vi "Teleop.vi"(10 "Match Info":T1={"Autonomous Elapsed Seconds"=0.0, "TeleOp Elapsed Seconds"=0.0, "Disabled Elapsed Seconds"=0.0, "Visited Autonomous"=FALSE, "Visited TeleOp"=FALSE, "Visited Disabled"=FALSE, "Autonomous Settings"={"Autonomous Style"=enum."Independent", "VI Refnum"=refnum}}, 11 "Call Context":T2) -> ()   [LabVIEW 2018]
doc: "This VI is called for each TeleOp packet received from the DS where the robot is not disabled. It is often used to read from the joysticks and update I/O or to update setpoints for timed control loops. It should complete and return within 20 milliseconds or it may miss DS packets."
uses:
  <vilib>/Rock Robotics/WPI/DriverStation/WPI_DriverStationDerivedRobotMode.ctl
  <vilib>/Rock Robotics/WPI/DriverStation/WPI_DriverStationMatch Info.ctl
  <vilib>/Rock Robotics/WPI/Solenoid/WPI_SolenoidValue.ctl
  <vilib>/Rock Robotics/WPI/ThirdParty/Phoenix-LabVIEW/Motor Controller/Controls/CTRE_Phoenix_MotorControl_ControlMode.ctl
  069bde93-6a50-4702-a448-63a100da85ba.vi
  93fe4f39-d887-44e8-b42b-40b0db67de57.vi
  <vilib>/Rock Robotics/WPI/Utilities/WPI_GetSetVariantRefNum.vi
  <vilib>/Rock Robotics/Network Tables/NT Write Boolean Array.vi
  <vilib>/Rock Robotics/Network Tables/NT Write Numeric Array.vi
  <vilib>/Rock Robotics/Network Tables/NT Read Boolean.vi
  <vilib>/Rock Robotics/Network Tables/NT Read Number.vi
  Robot Global Data.vi
  <vilib>/Rock Robotics/WPI/Solenoid/WPI_SolenoidSetEnum.vi
  <vilib>/Rock Robotics/WPI/ThirdParty/Phoenix-LabVIEW/Motor Controller/Get/CTRE_Phoenix_MotorController_GetSelectedSensorData.vi
  <vilib>/Rock Robotics/WPI/ThirdParty/Phoenix-LabVIEW/Motor Controller/Get/CTRE_Phoenix_MotorController_GetOutputCurrent_Enhanced.vi
panel:
  out "Level":string="Low"
  out "GamePiece":string="Hatch"
  out "Output Voltage 4":dbl
  out "Output Voltage 3":dbl
  out "Output Voltage 2":dbl
  out "Output Voltage":dbl
  out "wrist sensor":i32
  out "Arm sensor":i32
  out "x output 2":dbl
  out "y output 2":dbl
  out "Sample Slider 0":dbl(slide) scale=0.0..5.0
  out "Sample Boolean 1":bool
  out "Sample Boolean 0":bool
  # "left"
  # "RIGHT"
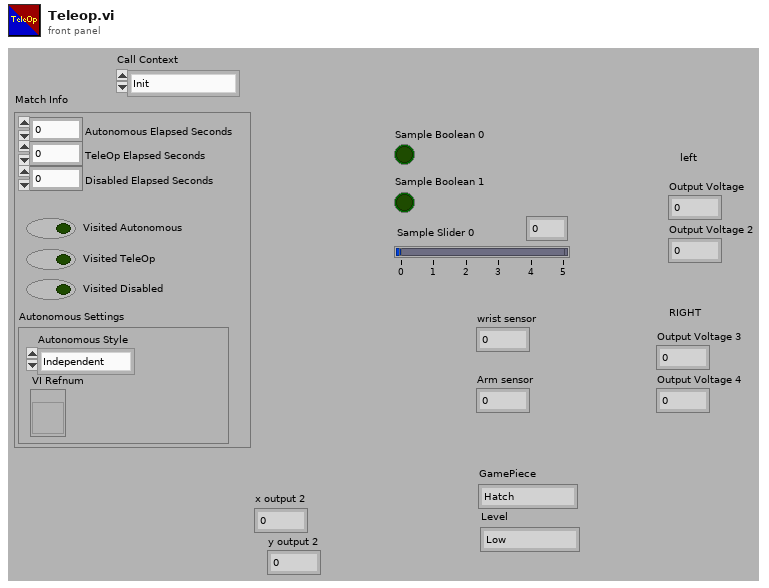
[diagram p1: front panel]
types:
  T1 = typedef "WPI_DriverStationMatch Info.ctl" = cluster{"Autonomous Elapsed Seconds":dbl, "TeleOp Elapsed Seconds":dbl, "Disabled Elapsed Seconds":dbl, "Visited Autonomous":bool, "Visited TeleOp":bool, "Visited Disabled":bool, "Autonomous Settings":cluster{"Autonomous Style":enum16{"Iterative", "Independent"}, "VI Refnum":refnum<vi>}}
  T2 = typedef "WPI_DriverStationDerivedRobotMode.ctl" = enum16{"Init", "Execute", "Stop"}
  T3 = typedef "WPI_SolenoidValue.ctl" = enum16{"Off", "On", "Forward", "Reverse"}
  T4 = typedef "WPI_JoystickDevRef.ctl" = cluster{"Device":T5}
  T5 = typedef "WPI_JoystickDeviceEnum.ctl" = enum16{"USB 0", "USB 1", "USB 2", "USB 3", "USB 4", "USB 5"}
  T6 = typedef "WPI_RobotDriveDevRef.ctl" = cluster{"DevStatus":errorcluster, "Motors[]":T7[], "Square Inputs":bool, "Max Output":dbl}
  T7 = typedef "WPI_MotorControlDeviceRef.ctl" = cluster{"DeviceStatus":errorcluster, "Type":T8, "PWM":cluster{"PWM Channel":T9, "DeadBand":T10}, "CAN":cluster{"Device Number":u8, "SetOutput VI Ref":variant, "GetOutput VI Ref":variant, "Enable VI Ref":variant, "Disable VI Ref":variant, "Data":variant}, "Invert":bool, "DIO PWM":cluster{"PWM \"Enable\" Channel":T9, "DIOChannel":T11, "PWM Rate":dbl}}
  T8 = typedef "WPI_MotorControlType.ctl" = enum16{"PWM", "CAN", "DIO PWM"}
  T9 = typedef "FPGA_DIOPWMChannel.ctl" = enum8{"PWM 0", "PWM 1", "PWM 2", "PWM 3", "PWM 4", "PWM 5", "PWM 6", "PWM 7", "PWM 8", "PWM 9", "PWM MXP 0", "PWM MXP 1", "PWM MXP 2", "PWM MXP 3", "PWM MXP 4", "PWM MXP 5", "PWM MXP 6", "PWM MXP 7", "PWM MXP 8", "PWM MXP 9", "Invalid"}
  T10 = typedef "WPI_PWMDeadband.ctl" = cluster{"Name":string, "maxPositivePwm":i32, "minPositivePwm":i32, "centerPwm":i32, "maxNegativePwm":i32, "minNegativePwm":i32, "angularRange":u16}
  T11 = typedef "FPGA_DIOChannel.ctl" = enum8{"DIO 0", "DIO 1", "DIO 2", "DIO 3", "DIO 4", "DIO 5", "DIO 6", "DIO 7", "DIO 8", "DIO 9", "DIO MXP 0", "DIO MXP 1", "DIO MXP 2", "DIO MXP 3", "DIO MXP 4", "DIO MXP 5", "DIO MXP 6", "DIO MXP 7", "DIO MXP 8", "DIO MXP 9", "DIO MXP 10", "DIO MXP 11", "DIO MXP 12", "DIO MXP 13", "DIO MXP 14", "DIO MXP 15", "SPI Port CS1", "SPI Port CS2", "SPI Port CS3", "SPI Port MISO", "SPI Port MOSI", "Invalid"}
  T12 = typedef "WPI_SolenoidDevRef.ctl" = cluster{"DevStatus":errorcluster, "Pneumatics Control Module":u8, "Forward Solenoid Channel":T13, "Reverse Solenoid Channel":T13}
  T13 = typedef "WPI_SolenoidChannel.ctl" = enum8{"Solenoid 0", "Solenoid 1", "Solenoid 2", "Solenoid 3", "Solenoid 4", "Solenoid 5", "Solenoid 6", "Solenoid 7", "Invalid"}
  T14 = typedef "CTRE_Phoenix_MotorControl_ControlMode.ctl" = u16
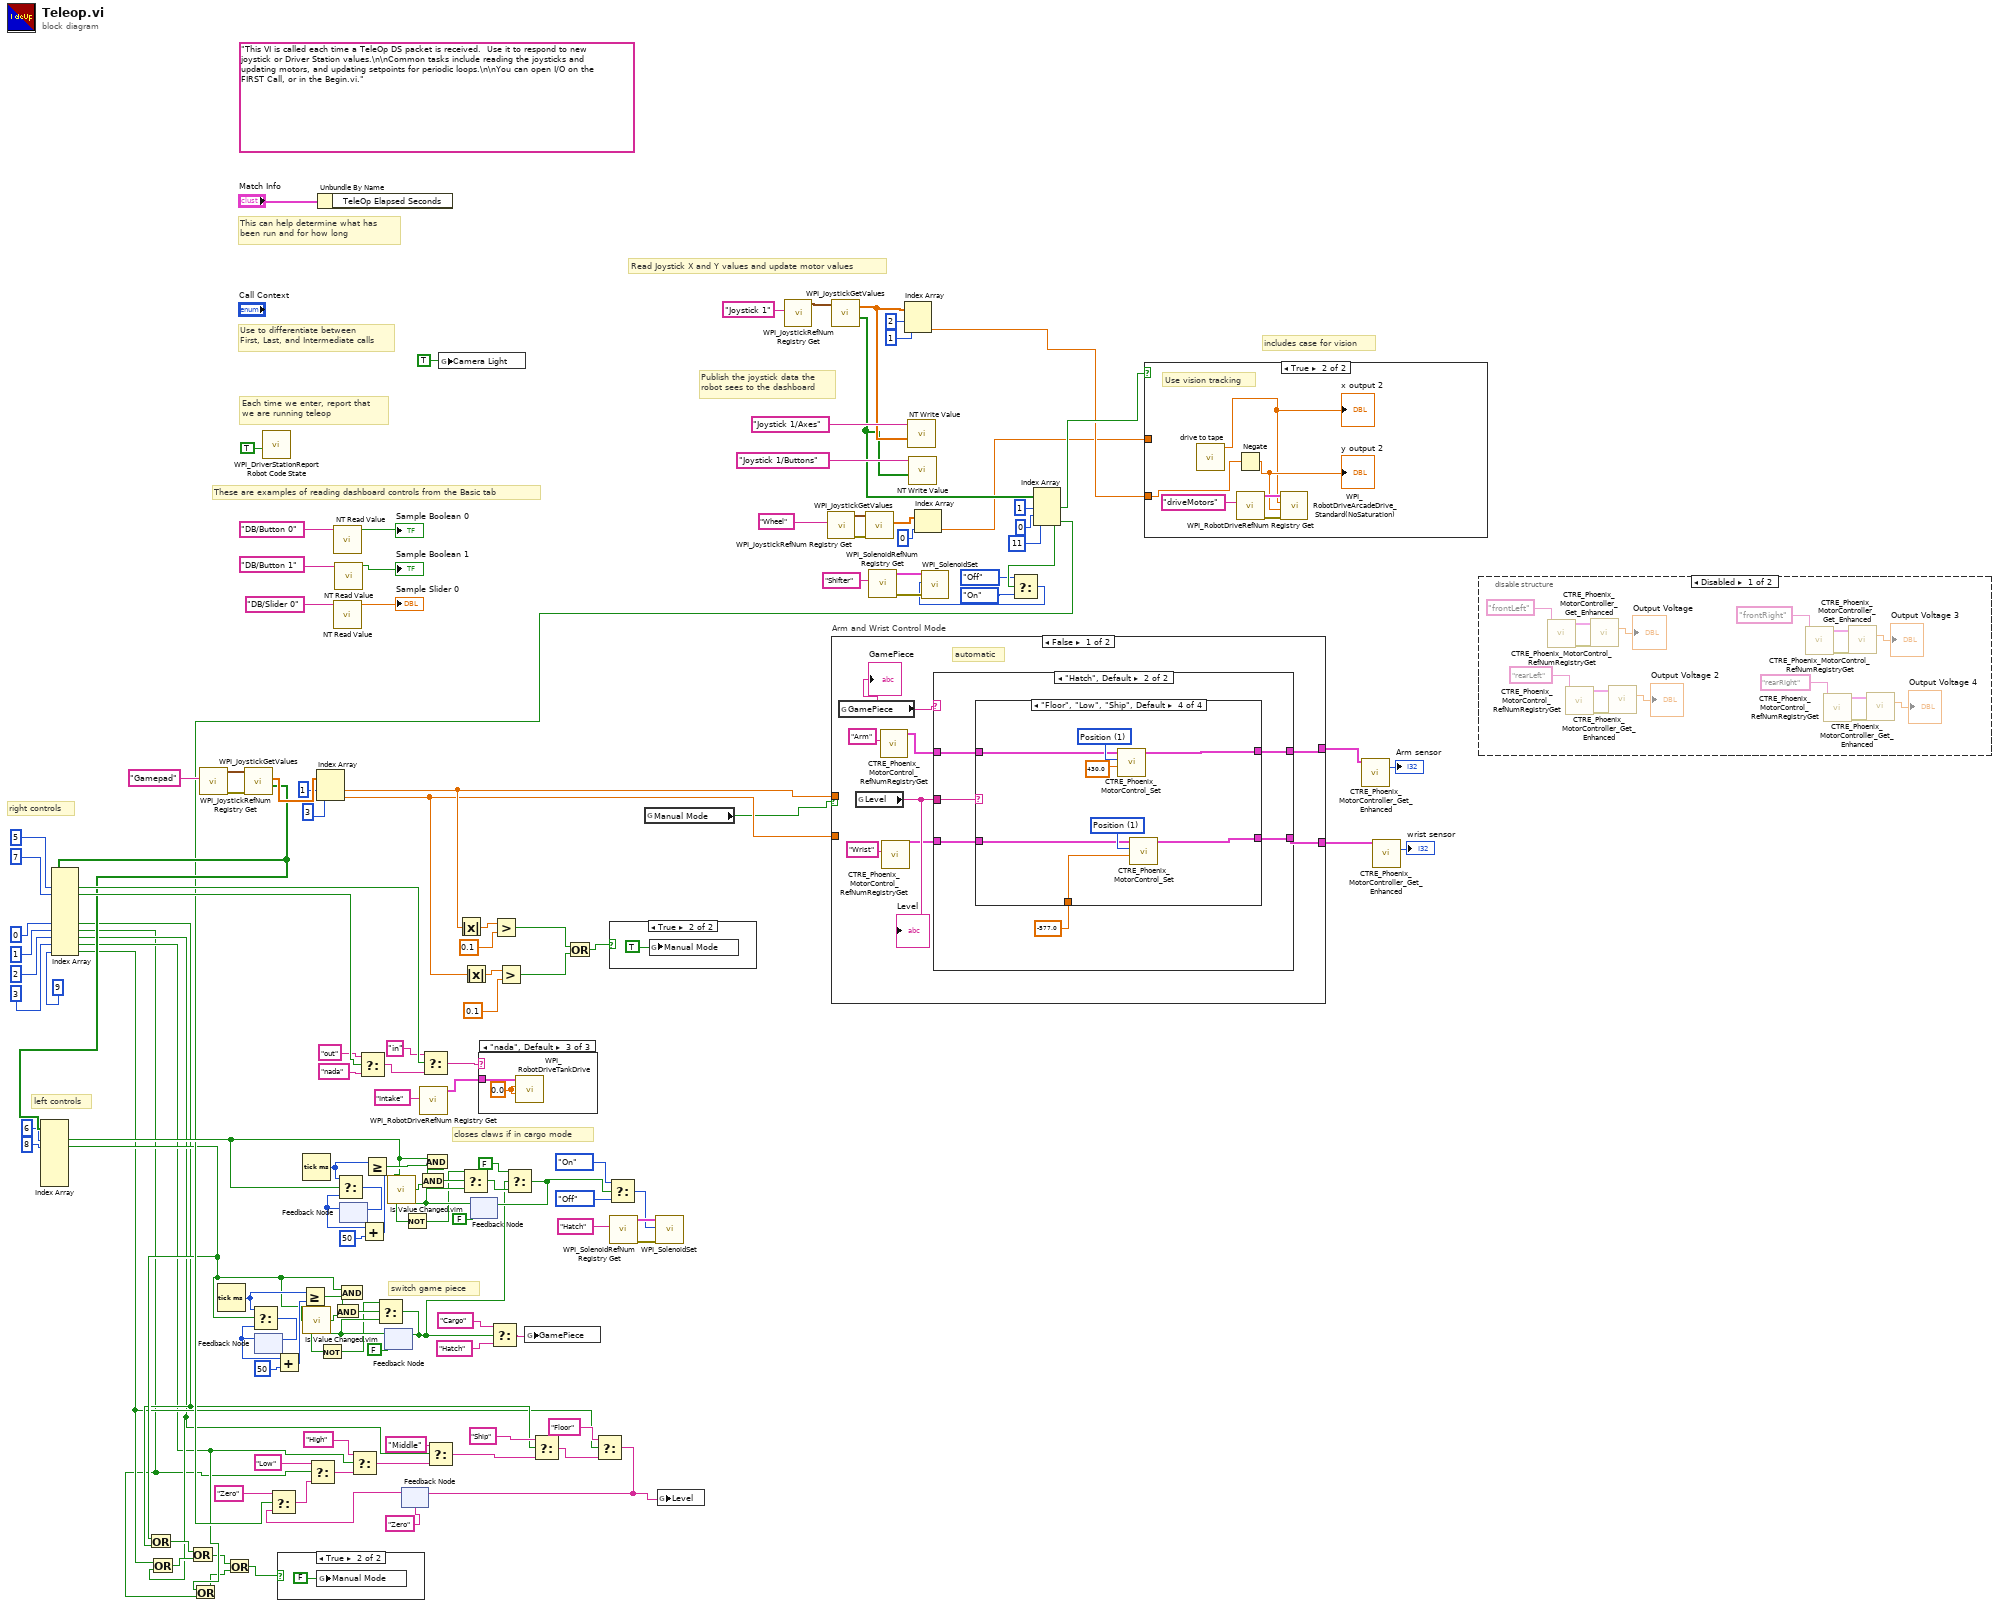
[diagram p0: block diagram]
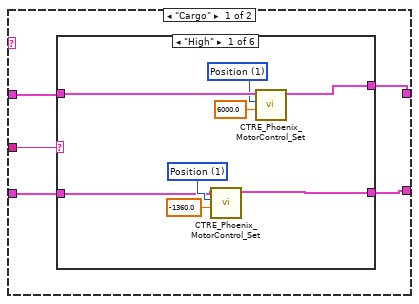
[diagram p5: hidden frame]
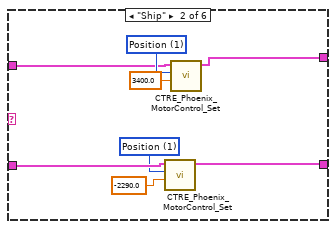
[diagram p6: hidden frame]
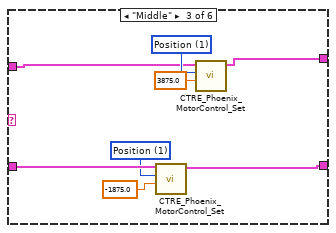
[diagram p7: hidden frame]
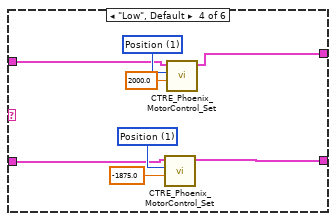
[diagram p8: hidden frame]
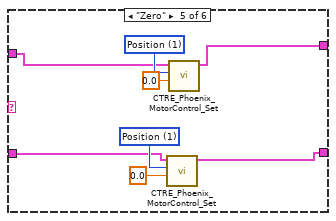
[diagram p9: hidden frame]
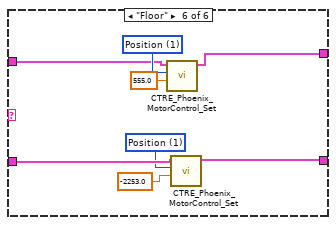
[diagram p10: hidden frame]
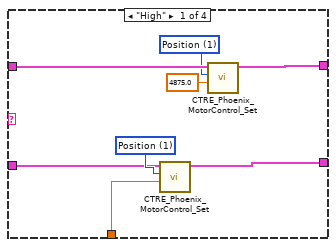
[diagram p11: hidden frame]
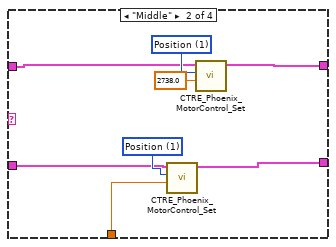
[diagram p12: hidden frame]
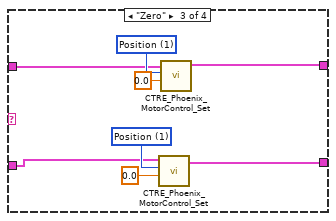
[diagram p13: hidden frame]
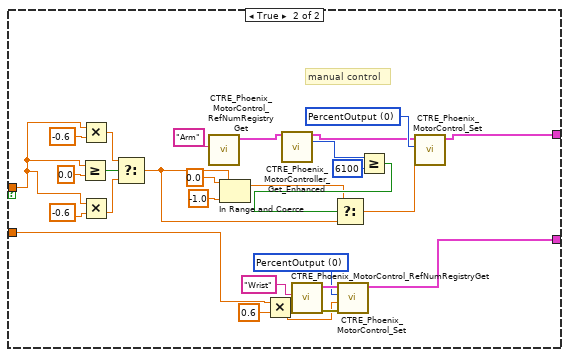
[diagram p14: hidden frame]
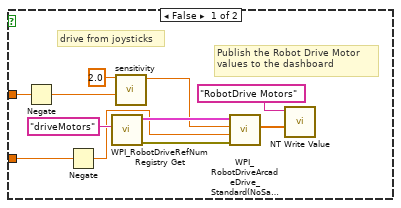
[diagram p15: hidden frame]
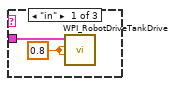
[diagram p16: hidden frame]
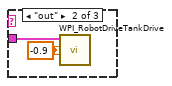
[diagram p17: hidden frame]
diagram:
  (unwired) "This VI is called each time a TeleOp DS packet is received.  Use it to respond to new joystick or Driver Station values.\n\nCommon tasks include reading the joysticks and updating motors, and updating setpoints for periodic loops.\n\nYou can open I/O on the FIRST Call, or in the Begin.vi."
  # "closes claws if in cargo mode"
  # "switch game piece"
  # "left controls"
  # "right controls"
  # "includes case for vision"
  # "These are examples of reading dashboard controls from the Basic tab"
  # "Publish the joystick data the\nrobot sees to the dashboard"
  # "Each time we enter, report that\nwe are running teleop"
  # "Use to differentiate between\nFirst, Last, and Intermediate calls"
  # "This can help determine what has\nbeen run and for how long"
  # "Read Joystick X and Y values and update motor values"
  n1 = call <vilib>:"WPI_JoystickRefNum Registry Get.vi"("refnum name"="Gamepad") -> ("error out"=w112:errorcluster, "JoystickDevRef"=w115:T4)  [unwired: 1 in, 8 out]
  n2 = Tick Count (ms)() -> (millisecond timer value=w62:u32)
  n3 = call <vilib>:"WPI_JoystickGetValues.vi"("error in (no error)"=w112, "JoystickDevRef"=w115) -> ("Buttons"=w36:bool[], "Axes"=w114:dbl[])  [unwired: 5 in, 3 out]
  n4 = Index Array(array=w36, index #1=6 ("index"), index #2=8 ("index")) -> (element #1=w33:bool, element #2=w9:bool)  [unwired: 5 in, 5 out]
  n5 = Index Array(array=w36, index #1=5 ("index"), index #2=7 ("index"), index #6=0 ("index"), index #7=1 ("index"), index #8=2 ("index"), index #9=3 ("index"), index #10=9 ("index")) -> (element #1=w109:bool, element #2=w104:bool, element #6=w8:bool, element #7=w4:bool, element #8=w6:bool, element #9=w5:bool, element #10=w7:bool)  [unwired: 3 in, 3 out]
  n6 = Or(x=w9, y=w8) -> (x .or. y?=w11:bool)
  n7 = Or(x=w7, y=w6) -> (x .or. y?=w10:bool)
  n8 = Or(x=w11, y=w10) -> (x .or. y?=w2:bool)
  n9 = Or(x=w5, y=w4) -> (x .or. y?=w3:bool)
  n10 = Or(x=w2, y=w3) -> (x .or. y?=w1:bool)
  n11 = feedback #1() -> (w53:u32)  [unwired: 1 in]
  n12 = Select(t=w62, s=w9, f=w53) -> (s? t:f=w60:u32)
  n13 = feedback-in #1(w60) -> ()
  n14 = call <vilib>:"WPI_DriverStationReport Robot Code State.vi"("TeleOp"=TRUE ("Autonomous")) -> ()  [unwired: 10 in, 1 out]
  n15 = Add(x=w53, y=u32 50) -> (x+y=w61:u32)
  n16 = case shown="True" w1 {
    frame False {
    }
    frame True {
      n17 = global write "Robot Global Data.vi" "Manual Mode"(FALSE) -> ()
    }
  }
  n18 = Greater Or Equal?(x=w62, y=w61) -> (x >= y?=w63:bool)
  n19 = Tick Count (ms)() -> (millisecond timer value=w79:u32)
  n20 = call "Is Value Changed.vim"("value"=w9) -> ("changed or first call?"=w58:bool)
  n21 = Index Array(array=w114, index #1=1 ("index"), index #2=3 ("index")) -> (element #1=w20:dbl, element #2=w15:dbl)
  n22 = Unbundle By Name("Match Info") -> ()  [unwired: 1 out]
  n23 = call-poly <vilib>:"NT Read Value.vi"("Name"="DB/Button 0" ("refnum name")) -> ("Boolean"=→"Sample Boolean 0":bool)  [unwired: 9 in, 1 out]
  n24 = call-poly <vilib>:"NT Read Value.vi"("Name"="DB/Slider 0" ("refnum name")) -> ("Numeric"=→"Sample Slider 0":dbl)  [unwired: 9 in, 1 out]
  n25 = call-poly <vilib>:"NT Read Value.vi"("Name"="DB/Button 1" ("refnum name")) -> ("Boolean"=→"Sample Boolean 1":bool)  [unwired: 9 in, 1 out]
  n26 = And(x=w9, y=w63) -> (x .and. y?=w64:bool)
  n27 = And(x=w64, y=w58) -> (x .and. y?=w57:bool)
  n28 = feedback #2() -> (w70:u32)  [unwired: 1 in]
  n29 = Select(t=w79, s=w33, f=w70) -> (s? t:f=w77:u32)
  n30 = feedback-in #2(w77) -> ()
  n31 = Select(t="out", s=w104, f="nada") -> (s? t:f=w105:string)
  n32 = Add(x=w70, y=u32 50) -> (x+y=w78:u32)
  n33 = Greater Or Equal?(x=w79, y=w78) -> (x >= y?=w80:bool)
  n34 = feedback #3(FALSE) -> (w56:bool)
  n35 = Not(x=w56) -> (.not. x?=w54:bool)
  n36 = Select(t=w54, s=w57, f=w56) -> (s? t:f=w24:bool)
  n37 = feedback-in #3(w24) -> ()
  n38 = call "Is Value Changed.vim"("value"=w33) -> ("changed or first call?"=w75:bool)
  n39 = feedback #4("Zero") -> (w30:string)
  n40 = call <vilib>:"WPI_RobotDriveRefNum Registry Get.vi"("refnum name"="Intake") -> ("RobotDriveDevRef"=w100:T6)  [unwired: 9 in, 1 out]
  n41 = Select(t="in", s=w109, f=w105) -> (s? t:f=w108:string)
  n42 = And(x=w33, y=w80) -> (x .and. y?=w81:bool)
  n43 = And(x=w81, y=w75) -> (x .and. y?=w74:bool)
  n44 = global write "Robot Global Data.vi" "Camera Light"(TRUE ("Camera Light")) -> ()
  n45 = Absolute Value(x=w20) -> (abs(x)=w22:dbl)
  n46 = Absolute Value(x=w15) -> (abs(x)=w18:dbl)
  n47 = feedback #5(FALSE) -> (w73:bool)
  n48 = Not(x=w73) -> (.not. x?=w71:bool)
  n49 = Select(t=w71, s=w74, f=w73) -> (s? t:f=w25:bool)
  n50 = case shown="\"nada\", Default" w108 {
    tunnel: w100 -> [w140 w142 w144]
    frame "in" {
      w141 = 0.8
      n51 = call <vilib>:"WPI_RobotDriveTankDrive.vi"("Right axis value"=w141, "Left axis value"=w141, "RobotDriveDevRef"=w140) -> ()  [unwired: 6 in, 3 out]
    }
    frame "out" {
      w143 = -0.9
      n52 = call <vilib>:"WPI_RobotDriveTankDrive.vi"("Right axis value"=w143, "Left axis value"=w143, "RobotDriveDevRef"=w142) -> ()  [unwired: 6 in, 3 out]
    }
    frame "nada", Default {
      w145 = 0.0
      n53 = call <vilib>:"WPI_RobotDriveTankDrive.vi"("Right axis value"=w145, "Left axis value"=w145, "RobotDriveDevRef"=w144) -> ()  [unwired: 6 in, 3 out]
    }
  }
  n54 = Select(t="Cargo", s=w24, f="Hatch") -> (s? t:f=w66:string)
  n55 = Greater?(x=w22, y=0.1) -> (0:w19:bool)
  n56 = Greater?(x=w18, y=0.1) -> (0:w16:bool)
  n57 = Select(t=FALSE, s=w24, f=w25) -> (s? t:f=w26:bool)
  n58 = feedback-in #5(w26) -> ()
  n59 = global write "Robot Global Data.vi" "GamePiece"(w66) -> ()
  n60 = Or(x=w19, y=w16) -> (x .or. y?=w13:bool)
  n61 = Select(t=WPI_SolenoidValue."On" ("Value"), s=w26, f=WPI_SolenoidValue."Off") -> (s? t:f=w96:T3)
  n62 = case shown="True" w13 {
    frame False {
    }
    frame True {
      n63 = global write "Robot Global Data.vi" "Manual Mode"(TRUE) -> ()
    }
  }
  n64 = call <vilib>:"WPI_SolenoidRefNum Registry Get.vi"("refnum name"="Hatch") -> ("error out"=w99:errorcluster, "SolenoidDevRef"=w98:T12)  [unwired: 9 in]
  n65 = global read "Robot Global Data.vi" "Manual Mode"() -> (w14:bool)
  n66 = call-poly <vilib>:"WPI_SolenoidSet.vi"("error in (no error)"=w99, "Value"=w96, "SolenoidDevRef"=w98) -> ()  [unwired: 7 in, 2 out]
  n67 = call <vilib>:"WPI_JoystickRefNum Registry Get.vi"("refnum name"="Joystick 1") -> ("JoystickDevRef"=w136:T4)  [unwired: 1 in, 9 out]
  n68 = call <vilib>:"WPI_JoystickRefNum Registry Get.vi"("refnum name"="Wheel") -> ("error out"=w123:errorcluster, "JoystickDevRef"=w122:T4)  [unwired: 9 in]
  n69 = call <vilib>:"WPI_JoystickGetValues.vi"("JoystickDevRef"=w136) -> ("Buttons"=w118:bool[], "Axes"=w132:dbl[])  [unwired: 6 in, 3 out]
  n70 = case "Arm and Wrist Control Mode" shown="False" w14 {
    tunnel: w15 -> [_ w266]
    tunnel: w20 -> [_ w258]
    tunnel: [w147 w257] -> w68
    tunnel: [w151 w256] -> w67
    frame False {
      # "automatic"
      n71 = global read "Robot Global Data.vi" "GamePiece"() -> (w150:string)
      "GamePiece" <- w150
      n72 = global read "Robot Global Data.vi" "Level"() -> (w149:string)
      "Level" <- w149
      n73 = call <vilib>:"CTRE_Phoenix_MotorControl_RefNumRegistryGet.vi"("refnum name"="Arm") -> ("PhoenixMotorControlDevRef"=w154:T7)  [unwired: 9 in, 1 out]
      n74 = call <vilib>:"CTRE_Phoenix_MotorControl_RefNumRegistryGet.vi"("refnum name"="Wrist") -> ("PhoenixMotorControlDevRef"=w148:T7)  [unwired: 9 in, 1 out]
      n75 = case shown="\"Hatch\", Default" w150 {
        tunnel: w154 -> [w158 w213]
        tunnel: [w159 w212] -> w151
        tunnel: [w157 w211] -> w147
        tunnel: w149 -> [w156 w210]
        tunnel: w148 -> [w155 w209]
        frame "Cargo" {
          n76 = case shown="\"High\"" w156 {
            tunnel: w158 -> [w167 w174 w182 w190 w195 w206]
            tunnel: [w165 w173 w181 w189 w194 w205] -> w159
            tunnel: [w163 w171 w179 w187 w193 w203] -> w157
            tunnel: w155 -> [w160 w170 w178 w184 w192 w202]
            frame "High" {
              w161 = T14 1 items=["PercentOutput"=0, "Position"=1, "Velocity"=2, "Current"=3, "Follower"=5, "MotionProfile"=6, "MotionMagic"=7, "MotionProfileArc"=10, "Disabled"=15] ("Control Mode")
              w166 = T14 1 items=["PercentOutput"=0, "Position"=1, "Velocity"=2, "Current"=3, "Follower"=5, "MotionProfile"=6, "MotionMagic"=7, "MotionProfileArc"=10, "Disabled"=15] ("Control Mode")
              n77 = call <vilib>:"CTRE_Phoenix_MotorControl_Set.vi"("Output"=-1360.0, "Control Mode"=w161, "PhoenixMotorControlDevRef"=w160) -> ("PhoenixMotorControlDevRef"=w163:T7)  [unwired: 7 in, 1 out]
              n78 = call <vilib>:"CTRE_Phoenix_MotorControl_Set.vi"("Output"=6000.0, "Control Mode"=w166, "PhoenixMotorControlDevRef"=w167) -> ("PhoenixMotorControlDevRef"=w165:T7)  [unwired: 7 in, 1 out]
            }
            frame "Ship" {
              w168 = T14 1 items=["PercentOutput"=0, "Position"=1, "Velocity"=2, "Current"=3, "Follower"=5, "MotionProfile"=6, "MotionMagic"=7, "MotionProfileArc"=10, "Disabled"=15] ("Control Mode")
              w175 = T14 1 items=["PercentOutput"=0, "Position"=1, "Velocity"=2, "Current"=3, "Follower"=5, "MotionProfile"=6, "MotionMagic"=7, "MotionProfileArc"=10, "Disabled"=15] ("Control Mode")
              n79 = call <vilib>:"CTRE_Phoenix_MotorControl_Set.vi"("Output"=-2290.0, "Control Mode"=w168, "PhoenixMotorControlDevRef"=w170) -> ("PhoenixMotorControlDevRef"=w171:T7)  [unwired: 7 in, 1 out]
              n80 = call <vilib>:"CTRE_Phoenix_MotorControl_Set.vi"("Output"=3400.0, "Control Mode"=w175, "PhoenixMotorControlDevRef"=w174) -> ("PhoenixMotorControlDevRef"=w173:T7)  [unwired: 7 in, 1 out]
            }
            frame "Middle" {
              w176 = T14 1 items=["PercentOutput"=0, "Position"=1, "Velocity"=2, "Current"=3, "Follower"=5, "MotionProfile"=6, "MotionMagic"=7, "MotionProfileArc"=10, "Disabled"=15] ("Control Mode")
              w183 = T14 1 items=["PercentOutput"=0, "Position"=1, "Velocity"=2, "Current"=3, "Follower"=5, "MotionProfile"=6, "MotionMagic"=7, "MotionProfileArc"=10, "Disabled"=15] ("Control Mode")
              n81 = call <vilib>:"CTRE_Phoenix_MotorControl_Set.vi"("Output"=-1875.0, "Control Mode"=w176, "PhoenixMotorControlDevRef"=w178) -> ("PhoenixMotorControlDevRef"=w179:T7)  [unwired: 7 in, 1 out]
              n82 = call <vilib>:"CTRE_Phoenix_MotorControl_Set.vi"("Output"=3875.0, "Control Mode"=w183, "PhoenixMotorControlDevRef"=w182) -> ("PhoenixMotorControlDevRef"=w181:T7)  [unwired: 7 in, 1 out]
            }
            frame "Low", Default {
              w185 = T14 1 items=["PercentOutput"=0, "Position"=1, "Velocity"=2, "Current"=3, "Follower"=5, "MotionProfile"=6, "MotionMagic"=7, "MotionProfileArc"=10, "Disabled"=15] ("Control Mode")
              w191 = T14 1 items=["PercentOutput"=0, "Position"=1, "Velocity"=2, "Current"=3, "Follower"=5, "MotionProfile"=6, "MotionMagic"=7, "MotionProfileArc"=10, "Disabled"=15] ("Control Mode")
              n83 = call <vilib>:"CTRE_Phoenix_MotorControl_Set.vi"("Output"=-1875.0, "Control Mode"=w185, "PhoenixMotorControlDevRef"=w184) -> ("PhoenixMotorControlDevRef"=w187:T7)  [unwired: 7 in, 1 out]
              n84 = call <vilib>:"CTRE_Phoenix_MotorControl_Set.vi"("Output"=2000.0, "Control Mode"=w191, "PhoenixMotorControlDevRef"=w190) -> ("PhoenixMotorControlDevRef"=w189:T7)  [unwired: 7 in, 1 out]
            }
            frame "Zero" {
              w196 = T14 1 items=["PercentOutput"=0, "Position"=1, "Velocity"=2, "Current"=3, "Follower"=5, "MotionProfile"=6, "MotionMagic"=7, "MotionProfileArc"=10, "Disabled"=15] ("Control Mode")
              w199 = T14 1 items=["PercentOutput"=0, "Position"=1, "Velocity"=2, "Current"=3, "Follower"=5, "MotionProfile"=6, "MotionMagic"=7, "MotionProfileArc"=10, "Disabled"=15] ("Control Mode")
              n85 = call <vilib>:"CTRE_Phoenix_MotorControl_Set.vi"("Output"=0.0, "Control Mode"=w196, "PhoenixMotorControlDevRef"=w192) -> ("PhoenixMotorControlDevRef"=w193:T7)  [unwired: 7 in, 1 out]
              n86 = call <vilib>:"CTRE_Phoenix_MotorControl_Set.vi"("Output"=0.0, "Control Mode"=w199, "PhoenixMotorControlDevRef"=w195) -> ("PhoenixMotorControlDevRef"=w194:T7)  [unwired: 7 in, 1 out]
            }
            frame "Floor" {
              w200 = T14 1 items=["PercentOutput"=0, "Position"=1, "Velocity"=2, "Current"=3, "Follower"=5, "MotionProfile"=6, "MotionMagic"=7, "MotionProfileArc"=10, "Disabled"=15] ("Control Mode")
              w207 = T14 1 items=["PercentOutput"=0, "Position"=1, "Velocity"=2, "Current"=3, "Follower"=5, "MotionProfile"=6, "MotionMagic"=7, "MotionProfileArc"=10, "Disabled"=15] ("Control Mode")
              n87 = call <vilib>:"CTRE_Phoenix_MotorControl_Set.vi"("Output"=555.0, "Control Mode"=w207, "PhoenixMotorControlDevRef"=w206) -> ("PhoenixMotorControlDevRef"=w205:T7)  [unwired: 7 in, 1 out]
              n88 = call <vilib>:"CTRE_Phoenix_MotorControl_Set.vi"("Output"=-2253.0, "Control Mode"=w200, "PhoenixMotorControlDevRef"=w202) -> ("PhoenixMotorControlDevRef"=w203:T7)  [unwired: 7 in, 1 out]
            }
          }
        }
        frame "Hatch", Default {
          n89 = case shown="\"Floor\", \"Low\", \"Ship\", Default" w210 {
            tunnel: w213 -> [w221 w228 w233 w244]
            tunnel: [w219 w227 w232 w243] -> w212
            tunnel: [w217 w225 w231 w241] -> w211
            tunnel: w209 -> [w215 w223 w230 w239]
            tunnel: -577.0 ("Output") -> [w214 w222 _ w238]
            frame "High" {
              w216 = T14 1 items=["PercentOutput"=0, "Position"=1, "Velocity"=2, "Current"=3, "Follower"=5, "MotionProfile"=6, "MotionMagic"=7, "MotionProfileArc"=10, "Disabled"=15] ("Control Mode")
              w220 = T14 1 items=["PercentOutput"=0, "Position"=1, "Velocity"=2, "Current"=3, "Follower"=5, "MotionProfile"=6, "MotionMagic"=7, "MotionProfileArc"=10, "Disabled"=15] ("Control Mode")
              n90 = call <vilib>:"CTRE_Phoenix_MotorControl_Set.vi"("Output"=w214, "Control Mode"=w216, "PhoenixMotorControlDevRef"=w215) -> ("PhoenixMotorControlDevRef"=w217:T7)  [unwired: 7 in, 1 out]
              n91 = call <vilib>:"CTRE_Phoenix_MotorControl_Set.vi"("Output"=4875.0, "Control Mode"=w220, "PhoenixMotorControlDevRef"=w221) -> ("PhoenixMotorControlDevRef"=w219:T7)  [unwired: 7 in, 1 out]
            }
            frame "Middle" {
              w224 = T14 1 items=["PercentOutput"=0, "Position"=1, "Velocity"=2, "Current"=3, "Follower"=5, "MotionProfile"=6, "MotionMagic"=7, "MotionProfileArc"=10, "Disabled"=15] ("Control Mode")
              w229 = T14 1 items=["PercentOutput"=0, "Position"=1, "Velocity"=2, "Current"=3, "Follower"=5, "MotionProfile"=6, "MotionMagic"=7, "MotionProfileArc"=10, "Disabled"=15] ("Control Mode")
              n92 = call <vilib>:"CTRE_Phoenix_MotorControl_Set.vi"("Output"=w222, "Control Mode"=w224, "PhoenixMotorControlDevRef"=w223) -> ("PhoenixMotorControlDevRef"=w225:T7)  [unwired: 7 in, 1 out]
              n93 = call <vilib>:"CTRE_Phoenix_MotorControl_Set.vi"("Output"=2738.0, "Control Mode"=w229, "PhoenixMotorControlDevRef"=w228) -> ("PhoenixMotorControlDevRef"=w227:T7)  [unwired: 7 in, 1 out]
            }
            frame "Zero" {
              w234 = T14 1 items=["PercentOutput"=0, "Position"=1, "Velocity"=2, "Current"=3, "Follower"=5, "MotionProfile"=6, "MotionMagic"=7, "MotionProfileArc"=10, "Disabled"=15] ("Control Mode")
              w237 = T14 1 items=["PercentOutput"=0, "Position"=1, "Velocity"=2, "Current"=3, "Follower"=5, "MotionProfile"=6, "MotionMagic"=7, "MotionProfileArc"=10, "Disabled"=15] ("Control Mode")
              n94 = call <vilib>:"CTRE_Phoenix_MotorControl_Set.vi"("Output"=0.0, "Control Mode"=w234, "PhoenixMotorControlDevRef"=w230) -> ("PhoenixMotorControlDevRef"=w231:T7)  [unwired: 7 in, 1 out]
              n95 = call <vilib>:"CTRE_Phoenix_MotorControl_Set.vi"("Output"=0.0, "Control Mode"=w237, "PhoenixMotorControlDevRef"=w233) -> ("PhoenixMotorControlDevRef"=w232:T7)  [unwired: 7 in, 1 out]
            }
            frame "Floor", "Low", "Ship", Default {
              w240 = T14 1 items=["PercentOutput"=0, "Position"=1, "Velocity"=2, "Current"=3, "Follower"=5, "MotionProfile"=6, "MotionMagic"=7, "MotionProfileArc"=10, "Disabled"=15] ("Control Mode")
              w245 = T14 1 items=["PercentOutput"=0, "Position"=1, "Velocity"=2, "Current"=3, "Follower"=5, "MotionProfile"=6, "MotionMagic"=7, "MotionProfileArc"=10, "Disabled"=15] ("Control Mode")
              n96 = call <vilib>:"CTRE_Phoenix_MotorControl_Set.vi"("Output"=430.0, "Control Mode"=w245, "PhoenixMotorControlDevRef"=w244) -> ("PhoenixMotorControlDevRef"=w243:T7)  [unwired: 7 in, 1 out]
              n97 = call <vilib>:"CTRE_Phoenix_MotorControl_Set.vi"("Output"=w238, "Control Mode"=w240, "PhoenixMotorControlDevRef"=w239) -> ("PhoenixMotorControlDevRef"=w241:T7)  [unwired: 7 in, 1 out]
            }
          }
        }
      }
    }
    frame True {
      w269 = T14 0 items=["PercentOutput"=0, "Position"=1, "Velocity"=2, "Current"=3, "Follower"=5, "MotionProfile"=6, "MotionMagic"=7, "MotionProfileArc"=10, "Disabled"=15] ("Control Mode")
      w273 = T14 0 items=["PercentOutput"=0, "Position"=1, "Velocity"=2, "Current"=3, "Follower"=5, "MotionProfile"=6, "MotionMagic"=7, "MotionProfileArc"=10, "Disabled"=15] ("Control Mode")
      # "manual control"
      n98 = Greater Or Equal?(x=w258, y=0.0) -> (x >= y?=w264:bool)
      n99 = Multiply(x=w258, y=-0.6) -> (x*y=w259:dbl)
      n100 = Multiply(x=w258, y=-0.6) -> (x*y=w263:dbl)
      n101 = Select(t=w259, s=w264, f=w263) -> (s? t:f=w250:dbl)
      n102 = call <vilib>:"CTRE_Phoenix_MotorControl_RefNumRegistryGet.vi"("refnum name"="Arm") -> ("PhoenixMotorControlDevRef"=w254:T7)  [unwired: 9 in, 1 out]
      n103 = In Range and Coerce(upper limit=0.0, x=w250, lower limit=-1.0) -> (coerced(x)=w246:dbl)  [unwired: 1 out]
      n104 = Multiply(x=w266, y=0.6) -> (x*y=w267:dbl)
      n105 = call-poly <vilib>:"CTRE_Phoenix_MotorController_Get_Enhanced.vi"("PhoenixMotorControlDevRef"=w254) -> ("PhoenixMotorControlDevRef"=w255:T7, "Position (Raw Sensor Units)"=w253:i32)  [unwired: 11 in, 2 out]
      n106 = call <vilib>:"CTRE_Phoenix_MotorControl_RefNumRegistryGet.vi"("refnum name"="Wrist") -> ("error out"=w271:errorcluster, "PhoenixMotorControlDevRef"=w270:T7)  [unwired: 9 in]
      n107 = call <vilib>:"CTRE_Phoenix_MotorControl_Set.vi"("error in (no error)"=w271, "Output"=w267, "Control Mode"=w269, "PhoenixMotorControlDevRef"=w270) -> ("PhoenixMotorControlDevRef"=w257:T7)  [unwired: 6 in, 1 out]
      n108 = Greater Or Equal?(x=w253, y=6100) -> (x >= y?=w251:bool)
      n109 = Select(t=w246, s=w251, f=w250) -> (s? t:f=w247:dbl)
      n110 = call <vilib>:"CTRE_Phoenix_MotorControl_Set.vi"("Output"=w247, "Control Mode"=w273, "PhoenixMotorControlDevRef"=w255) -> ("PhoenixMotorControlDevRef"=w256:T7)  [unwired: 7 in, 1 out]
    }
  }
  n111 = call <vilib>:"WPI_JoystickGetValues.vi"("error in (no error)"=w123, "JoystickDevRef"=w122) -> ("Axes"=w121:dbl[])  [unwired: 5 in, 4 out]
  n112 = call <vilib>:"WPI_SolenoidRefNum Registry Get.vi"("refnum name"="Shifter") -> ("error out"=w92:errorcluster, "SolenoidDevRef"=w91:T12)  [unwired: 9 in]
  n113 = Index Array(array=w132, index #1=2 ("index"), index #2=1 ("index")) -> (element #2=w83:dbl)  [unwired: 1 out]
  n114 = call-poly <vilib>:"NT Write Value.vi"("Numeric Array"=w132, "Name"="Joystick 1/Axes") -> ()  [unwired: 9 in, 1 out]
  n115 = call-poly <vilib>:"NT Write Value.vi"("Boolean Array"=w118, "Name"="Joystick 1/Buttons") -> ()  [unwired: 9 in, 1 out]
  n116 = Index Array(array=w121, index=0) -> (element=w82:dbl)
  n117 = Index Array(array=w118, index #1=1 ("index"), index #2=0 ("index"), index #3=11 ("index")) -> (element #1=w84:bool, element #2=w89:bool, element #3=w12:bool)
  n118 = Select(t="Zero", s=w12, f=w30) -> (s? t:f=w27:string)
  n119 = Select(t="Low", s=w4, f=w27) -> (s? t:f=w44:string)
  n120 = Select(t="High", s=w5, f=w44) -> (s? t:f=w43:string)
  n121 = Select(t="Middle", s=w6, f=w43) -> (s? t:f=w41:string)
  n122 = Select(t="Ship", s=w8, f=w41) -> (s? t:f=w37:string)
  n123 = Select(t="Floor", s=w7, f=w37) -> (s? t:f=w39:string)
  n124 = feedback-in #4(w39) -> ()
  n125 = global write "Robot Global Data.vi" "Level"(w39) -> ()
  n126 = Select(t=WPI_SolenoidValue."Off" ("Value"), s=w89, f=WPI_SolenoidValue."On" ("Value")) -> (s? t:f=w88:T3)
  n127 = call-poly <vilib>:"WPI_SolenoidSet.vi"("error in (no error)"=w92, "Value"=w88, "SolenoidDevRef"=w91) -> ()  [unwired: 7 in, 2 out]
  n128 = case shown="True" w84 {
    tunnel: w83 -> [w280 w285]
    tunnel: w82 -> [w279 _]
    frame False {
      # "drive from joysticks"
      # "Publish the Robot Drive Motor\nvalues to the dashboard"
      n129 = Negate(x=w279) -> (-x=w276:dbl)
      n130 = Negate(x=w280) -> (-x=w277:dbl)
      n131 = call <vilib>:"WPI_RobotDriveRefNum Registry Get.vi"("refnum name"="driveMotors") -> ("error out"=w278:errorcluster, "RobotDriveDevRef"=w283:T6)  [unwired: 1 in, 8 out]
      n132 = call "sensitivity.vi"("x"=w276, "sensitivity"=2.0) -> ("scaled value"=w275:dbl)  [unwired: 9 in]
      n133 = call <vilib>:"WPI_RobotDriveArcadeDrive_Standard(NoSaturation).vi"("error in (no error)"=w278, "Y axis value"=w277, "X axis value"=w275, "RobotDriveDevRef"=w283) -> ("Motor Values"=w284:dbl[])  [unwired: 7 out]
      n134 = call-poly <vilib>:"NT Write Value.vi"("Numeric Array"=w284, "Name"="RobotDrive Motors") -> ()  [unwired: 9 in, 1 out]
    }
    frame True {
      # "Use vision tracking"
      n135 = call "drive to tape.vi"() -> ("x output"=w286:dbl)  [unwired: 10 in, 1 out]
      "x output 2" <- w286
      n136 = Negate(x=w285) -> (-x=w287:dbl)
      "y output 2" <- w287
      n137 = call <vilib>:"WPI_RobotDriveRefNum Registry Get.vi"("refnum name"="driveMotors") -> ("error out"=w288:errorcluster, "RobotDriveDevRef"=w289:T6)  [unwired: 1 in, 8 out]
      n138 = call <vilib>:"WPI_RobotDriveArcadeDrive_Standard(NoSaturation).vi"("error in (no error)"=w288, "Y axis value"=w287, "X axis value"=w286, "RobotDriveDevRef"=w289) -> ()  [unwired: 8 out]
    }
  }
  n139 = call-poly <vilib>:"CTRE_Phoenix_MotorController_Get_Enhanced.vi"("PhoenixMotorControlDevRef"=w67) -> ("Position (Raw Sensor Units)"=→"Arm sensor":i32)  [unwired: 11 in, 3 out]
  n140 = call-poly <vilib>:"CTRE_Phoenix_MotorController_Get_Enhanced.vi"("PhoenixMotorControlDevRef"=w68) -> ("Position (Raw Sensor Units)"=→"wrist sensor":i32)  [unwired: 11 in, 3 out]
  n141 = disable-structure shown="Disabled" {
    frame Disabled {
      n142 = call <vilib>:"CTRE_Phoenix_MotorControl_RefNumRegistryGet.vi"("refnum name"="frontLeft") -> ("error out"=w305:errorcluster, "PhoenixMotorControlDevRef"=w306:T7)  [unwired: 9 in]
      n143 = call <vilib>:"CTRE_Phoenix_MotorControl_RefNumRegistryGet.vi"("refnum name"="rearLeft") -> ("error out"=w302:errorcluster, "PhoenixMotorControlDevRef"=w303:T7)  [unwired: 9 in]
      n144 = call-poly <vilib>:"CTRE_Phoenix_MotorController_Get_Enhanced.vi"("PhoenixMotorControlDevRef"=w306, "error in"=w305) -> ("Output Current"=→"Output Voltage":dbl)  [unwired: 11 in, 2 out]
      n145 = call-poly <vilib>:"CTRE_Phoenix_MotorController_Get_Enhanced.vi"("PhoenixMotorControlDevRef"=w303, "error in"=w302) -> ("Output Current"=→"Output Voltage 2":dbl)  [unwired: 11 in, 2 out]
      n146 = call <vilib>:"CTRE_Phoenix_MotorControl_RefNumRegistryGet.vi"("refnum name"="frontRight") -> ("error out"=w299:errorcluster, "PhoenixMotorControlDevRef"=w300:T7)  [unwired: 9 in]
      n147 = call <vilib>:"CTRE_Phoenix_MotorControl_RefNumRegistryGet.vi"("refnum name"="rearRight") -> ("error out"=w296:errorcluster, "PhoenixMotorControlDevRef"=w297:T7)  [unwired: 9 in]
      n148 = call-poly <vilib>:"CTRE_Phoenix_MotorController_Get_Enhanced.vi"("PhoenixMotorControlDevRef"=w300, "error in"=w299) -> ("Output Current"=→"Output Voltage 3":dbl)  [unwired: 11 in, 2 out]
      n149 = call-poly <vilib>:"CTRE_Phoenix_MotorController_Get_Enhanced.vi"("PhoenixMotorControlDevRef"=w297, "error in"=w296) -> ("Output Current"=→"Output Voltage 4":dbl)  [unwired: 11 in, 2 out]
    }
    frame Enabled {
    }
  }
